vi "Z6_Beamline.set Switch State in GUI.vi"(0 "i ref in":refnum<vi>, 1 "Boolean GUI Ref":refnum<vi>, 2 "Pic GUI Ref":refnum<vi>, 3 "Status":T1 items=["no info", "off/false/out", "on/true/in", "Failure", "Alarm", "Status 1", "Status 2", "Status 3"], 4 "no Link?":bool, 5 "error in (no error)":errorcluster) -> (14 "i ref out":refnum<vi>, 19 "error out":errorcluster)   [LabVIEW 2014, in "Z6_Beamline.lvlib"]
doc: "This VI writes the incoming information about switches to the GUI."
uses:
  Z6_Beamline.lvlib
  PH_StatusHandler/PH_StatusHandler.Status.ctl
  PH_BL-Master/PH_BL-Master.Shutter State.ctl
  PH_Beamline/PH_Beamline.Switch Instances.ctl
  PH_Common/PH_Common.lvlib
  PH_StatusHandler/PH_StatusHandler.lvlib
  PH_Beamline/PH_Beamline.lvlib
  PH_Switch/PH_Switch.lvlib
  PH_Beamline_Common/PH_Beamline_Common.lvlib
  PH_BL-Master/PH_BL-Master.lvlib
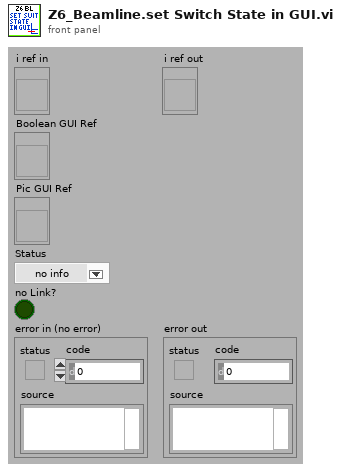
[diagram p1: front panel]
types:
  T1 = typedef "PH_StatusHandler.lvlib/PH_StatusHandler.Status.ctl" = i16
  T2 = typedef "PH_BL-Master.lvlib/PH_BL-Master.Shutter State.ctl" = enum16{"No Link", "No Info", "In", "Out", "in between"}
  T3 = typedef "PH_Beamline.lvlib/PH_Beamline.Switch Instances.ctl" = string
  T4 = enum16{"No Link", "No Info", "In", "Out", "in between"}
  T5 = typedef "Z6_Beamline.lvlib/Z6_Beamline.i attribute.ctl" = cluster{"Subs ok GUI Refs":T6, "Refs BL Northtower":refnum<vi>[], "Refs BL Southtower":refnum<vi>[], "Refs BL 100TW COS":refnum<vi>[], "State Subsystems":cluster{"Northtower":bool, "Southtower":bool, "Frontends":bool, "100TW COS":bool}, "Z6 Beamline Status Subscriber Information":T7, "Color State PHELIX":i16}
  T6 = typedef "Z6_Beamline.lvlib/Z6_Beamline.Subsystem ok GUI Refs.ctl" = cluster{"Northtower ok":refnum<vi>, "Southtower ok":refnum<vi>, "Frontends ok":refnum<vi>, "100TW COS ok":refnum<vi>}
  T7 = typedef "Z6_Beamline.lvlib/Z6_Beamline.Status Subscriber Information.ctl" = cluster{"BL Z6 Shutter":T8, "CH 10":T8, "CH 11":T8, "ST Flip Cam":T8, "ST Flip DB":T8, "BL Z6 Dump":T8}
  T8 = typedef "PH_BL-Master.lvlib/PH_BL-Master.Status Subscriber Information.ctl" = cluster{"Index of element":i32, "Attributeset":T9}
  T9 = typedef "PH_BL-Master.lvlib/PH_BL-Master.Attribute Set.ctl" = enum16{"Boolean Status Service Subscriber", "Picture Status Service Subscriber"}
  T10 = typedef "PH_BL-Master.lvlib/PH_BL-Master.i attribute.ctl" = cluster{"Remote controlled":bool, "Boolean Condition Service Subscriber":refnum<vi>[], "Picture Condition Service Subscriber":refnum<vi>[], "R2S":cluster{"GUI Ref":refnum<vi>, "State":bool}, "Vacua":cluster{"GUI Ref":refnum<vi>, "Limit":dbl, "Curr Value":dbl, "in range":bool}[], "O2 Inspection":cluster{"GUI Ref":refnum<vi>, "Concentration":dbl, "State":T1}[], "Boolean Status Service Subscriber":cluster{"GUI Ref":refnum<vi>, "Status":T1, "no Link?":bool, "Status Subscriber Class":T11}[], "Picture Status Service Subscriber":cluster{"GUI Ref":refnum<vi>, "Status":T1, "no Link?":bool, "Status Subscriber Class":T11}[], "6P 4Q Service Subscriber":cluster{"GUI Ref":refnum<vi>, "Selector":T12, "no Link?":bool}[], "Index of latest 6P 4Q changing Instance":i32, "Index of latest Picture Status changing Instance":i32, "Index of latest Boolean Status changing Instance":i32, "Vision ID on same Node":string, "Start Phase over?":bool, "GUI Ref Delete":refnum<vi>}
  T11 = typedef "PH_BL-Master.lvlib/PH_BL-Master.Status Subscriber Class.ctl" = enum16{"unknown", "Switch", "BB", "6P Switch", "Switch GUI", "Switch and 6P State", "Force Sensor"}
  T12 = typedef "PH_4_Pos_Selector.lvlib/PH_4_Pos_Selector.Position Selector.ctl" = u16
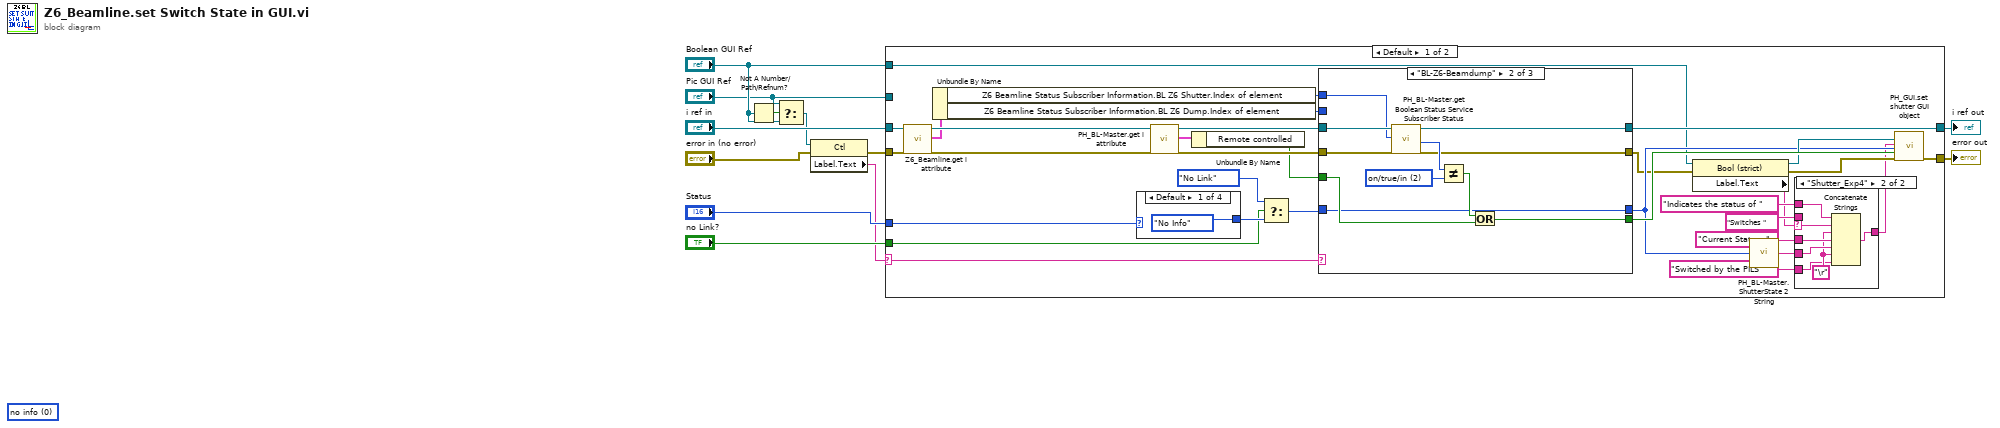
[diagram p0: block diagram]
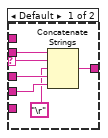
[diagram p2: hidden frame]
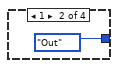
[diagram p3: hidden frame]
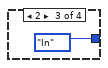
[diagram p4: hidden frame]
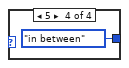
[diagram p5: hidden frame]
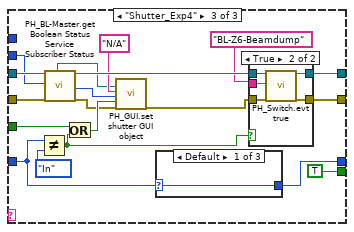
[diagram p7: hidden frame]
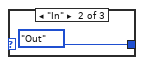
[diagram p8: hidden frame]
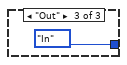
[diagram p9: hidden frame]
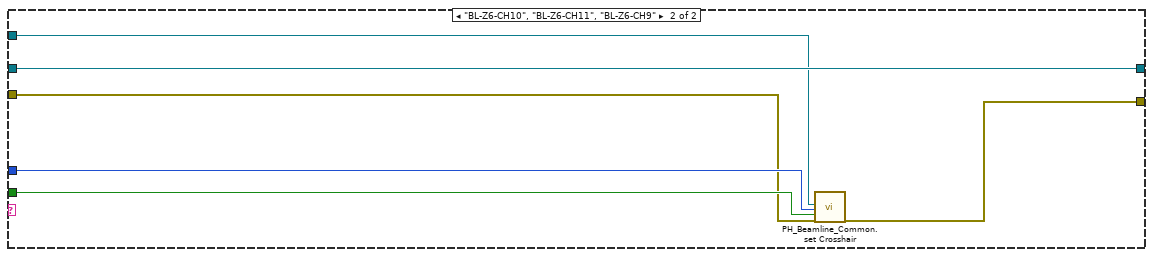
[diagram p11: hidden frame]
diagram:
  (unwired) T1 0 items=["no info", "off/false/out", "on/true/in", "Failure", "Alarm", "Status 1", "Status 2", "Status 3"] ("Status")
  n1 = Not A Number/Path/Refnum?(number/path/refnum="Boolean GUI Ref") -> (NaN/Path/Refnum?=w6:bool)
  n2 = Select(t="Pic GUI Ref", s=w6, f="Boolean GUI Ref") -> (s? t:f=w7:refnum<vi>)
  n3 = property class="Ctl"(reference=w7, error in="error in (no error)") -> (error out=w4:errorcluster, "Label.Text"=w1:string)  [unwired: 1 out]
  n4 = case "Empty Name, Crosshairs and normal Switches ..." shown="Default" w1 {
    selector: w1 -> [w43 _]
    tunnel: w4 -> [w22 w106]
    tunnel: "i ref in" -> [w18 w110]
    tunnel: "Status" -> [w29 w109]
    tunnel: "no Link?" -> [w28 w108]
    tunnel: [w44 w111] -> w11
    tunnel: [w42 w110] -> w10
    tunnel: "Boolean GUI Ref" -> [w26 _]
    tunnel: "Pic GUI Ref" -> [_ w107]
    frame Default {
      n5 = call "Z6_Beamline.get i attribute.vi"("i ref in"=w18, "error in (no error)"=w22) -> ("i ref out"=w17:refnum<vi>, "i attribute"=w16:T5, "error out"=w19:errorcluster)  [unwired: 15 in]
      n6 = Unbundle By Name(w16) -> ("Z6 Beamline Status Subscriber Information.BL Z6 Shutter.Index of element"=w14:i32, "Z6 Beamline Status Subscriber Information.BL Z6 Dump.Index of element"=w15:i32)
      n7 = case shown="Default" w29 {
        tunnel: [PH_BL-Master.Shutter_State."No Info" ("Shutter State") PH_BL-Master.Shutter_State."Out" ("Shutter State") PH_BL-Master.Shutter_State."In" ("Shutter State") PH_BL-Master.Shutter_State."in between" ("Shutter State")] -> w30
        frame Default {
        }
        frame 1 {
        }
        frame 2 {
        }
        frame 5 {
        }
      }
      n8 = call "PH_BL-Master.get i attribute.vi"("i ref in"=w17, "error in (no error)"=w19) -> ("i ref out"=w20:refnum<vi>, "i attribute"=w23:T10, "error out"=w21:errorcluster)  [unwired: 15 in]
      n9 = Unbundle By Name(w23) -> ("Remote controlled"=w13:bool)
      n10 = Select(t=PH_BL-Master.Shutter_State."No Link" ("Shutter State"), s=w28, f=w30) -> (s? t:f=w27:T2)
      n11 = case shown="\"BL-Z6-Beamdump\"" w43 {
        tunnel: w13 -> [w65 w69 w93]
        tunnel: [w65 w75 TRUE] -> w41
        tunnel: w20 -> [w64 w72 w90]
        tunnel: [w64 w71 w87] -> w42
        tunnel: w21 -> [w63 w70 w91]
        tunnel: [w63 w68 w88] -> w24
        tunnel: w27 -> [w62 w67 w84]
        tunnel: [w62 w67 w83] -> w33
        tunnel: w15 -> [_ _ w77]
        tunnel: w14 -> [_ w66 _]
        frame Default {
        }
        frame "BL-Z6-Beamdump" {
          w76 = T1 2 items=["no info", "off/false/out", "on/true/in", "Failure", "Alarm", "Status 1", "Status 2", "Status 3"] ("State")
          n12 = call "PH_BL-Master.get Boolean Status Service Subscriber Status.vi"("i ref in"=w72, "Index of wanted element"=w66, "error in (no error)"=w70) -> ("i ref out"=w71:refnum<vi>, "Subscriber State"=w73:T1, "error out"=w68:errorcluster)  [unwired: 8 in, 6 out]
          n13 = Not Equal?(x=w73, y=w76) -> (x != y?=w74:bool)
          n14 = Or(x=w74, y=w69) -> (x .or. y?=w75:bool)
        }
        frame "Shutter_Exp4" {
          n15 = Not Equal?(x=w84, y=PH_BL-Master.Shutter_State."In" ("State")) -> (x != y?=w82:bool)
          n16 = call "PH_BL-Master.get Boolean Status Service Subscriber Status.vi"("i ref in"=w90, "Index of wanted element"=w77, "error in (no error)"=w91) -> ("Wanted Boolean Ref"=w78:refnum<vi>, "i ref out"=w86:refnum<vi>, "Subscriber State"=w89:T1, "error out"=w79:errorcluster)  [unwired: 8 in, 5 out]
          n17 = Or(x=w93, y=w82) -> (x .or. y?=w92:bool)
          n18 = call "PH_GUI.set shutter GUI object.vi"("Wanted Boolean Ref"=w78, "Tip Strip"="N/A", "Shutter State"=w89, "Disabled? (false)"=w92, "error in (no error)"=w79) -> ("error out"=w85:errorcluster)  [unwired: 14 in]
          n19 = case shown="Default" w84 {
            selector: w84 -> [w96 _ _]
            tunnel: [w96 T4."Out" ("Shutter State") T4."In" ("Shutter State")] -> w83
            frame Default {
            }
            frame "In" {
            }
            frame "Out" {
            }
          }
          n20 = case shown="True" w82 {
            tunnel: [w99 w105] -> w88
            tunnel: [w100 w104] -> w87
            tunnel: w86 -> [w100 w103]
            tunnel: w85 -> [w99 w102]
            tunnel: T3 "BL-Z6-Beamdump" ("Switch Instance") -> [_ w101]
            frame False {
            }
            frame True {
              n21 = call "PH_Switch.evt true.vi"("i ref in"=w103, "Instance"=w101, "error in (no error)"=w102) -> ("i ref out"=w104:refnum<vi>, "error out"=w105:errorcluster)  [unwired: 15 in]
            }
          }
        }
      }
      n22 = property class="Bool (strict)"(reference=w26, error in=w24) -> (reference out=w35:refnum<vi>, error out=w34:errorcluster, "Label.Text"=w25:string)
      n23 = call "PH_BL-Master.ShutterState 2 String.vi"("Shutter State"=w33) -> ("String"=w36:string)
      n24 = case shown="\"Shutter_Exp4\"" w25 {
        selector: w25 -> [w45 w54]
        tunnel: [w50 w57] -> w32
        tunnel: "Current Status: " ("string") -> [w49 w56]
        tunnel: w36 -> [w48 w55]
        tunnel: "Switches " ("string") -> [w46 _]
        tunnel: "Indicates the status of " ("string") -> [_ w53]
        tunnel: "Switched by the PILS" ("string") -> [_ w51]
        frame Default {
          n25 = Concatenate Strings(w46, w45, "\r", w49, w48) -> (w50:string)
        }
        frame "Shutter_Exp4" {
          w52 = "\r"
          n26 = Concatenate Strings(w53, w54, w52, w56, w55, w52, w51) -> (w57:string)
        }
      }
      n27 = call "PH_GUI.set shutter GUI object.vi"("Wanted Boolean Ref"=w35, "Tip Strip"=w32, "Shutter State"=w33, "Disabled? (false)"=w41, "error in (no error)"=w34) -> ("error out"=w44:errorcluster)  [unwired: 14 in]
    }
    frame "BL-Z6-CH10", "BL-Z6-CH11", "BL-Z6-CH9" {
      n28 = call "PH_Beamline_Common.set Crosshair.vi"("CtlRef"=w107, "State"=w109, "no link"=w108, "error in (no error)"=w106) -> ("error out"=w111:errorcluster)  [unwired: 15 in]
    }
  }
  "error out" <- w11
  "i ref out" <- w10
